vi "Containers by Target.vi"(7 "Target Name":string, 10 "Targets":refnum<vi>[](array[refnum])) -> (1 "Container Names":string[](array[string]), 2 "Container Paths":path[](array[path]), 3 "Target":refnum<vi>)   [LabVIEW 2020, in "Conditum-Tools.lvlib" / "Entity Editor.lvclass"]
uses:
  Entity Editor.lvclass
  Entity Editor.lvclass/Entity Editor.ctl
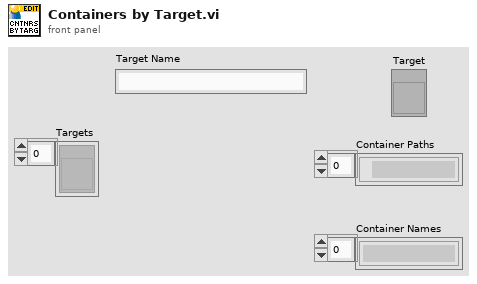
[diagram p1: front panel]
types:
  T1 = enum32{"invalid scope", "public", "private", "protected", "community"}
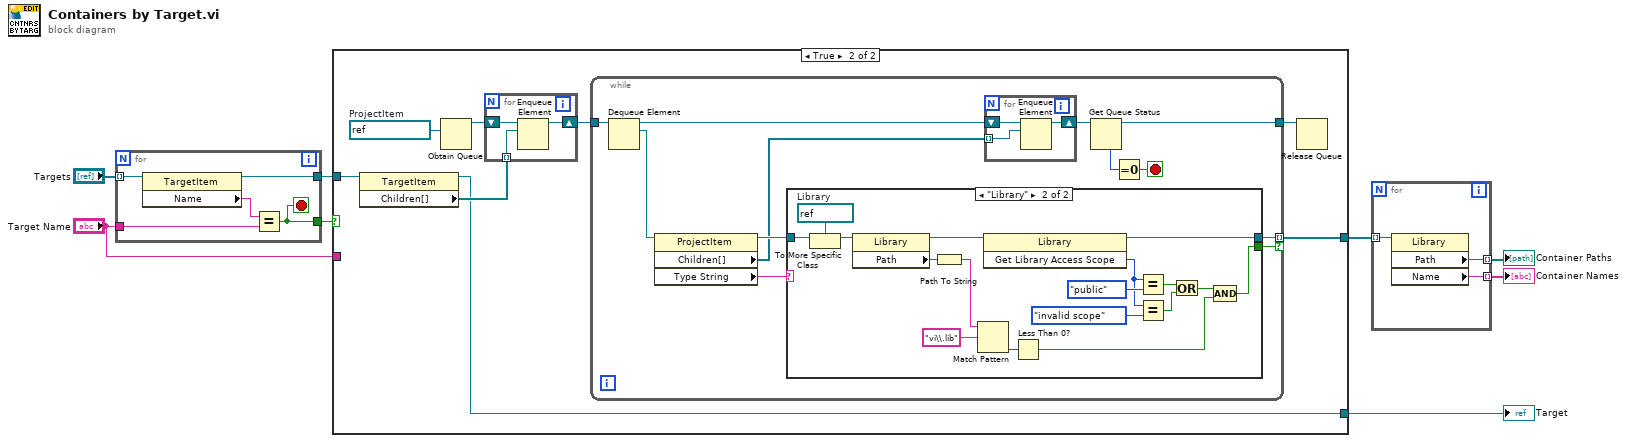
[diagram p0: block diagram]
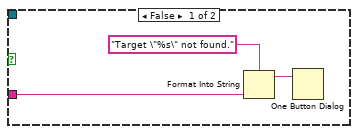
[diagram p2: hidden frame]
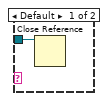
[diagram p3: hidden frame]
diagram:
  n1 = for {
    tunnel: "Targets" -> [w13] mode=indexing
    tunnel: "Target Name" -> [w12]
    tunnel: [w10] -> w6
    tunnel: [w9] -> w7
    stop <- w9 stop-if-true
    n2 = property class="TargetItem"(reference=w13) -> (reference out=w10:refnum<vi>, "Name"=w11:string)  [unwired: 1 in, 1 out]
    n3 = Equal?(x=w11, y=w12) -> (x = y?=w9:bool)
  }
  n4 = case shown="True" w7 {
    tunnel: w6 -> [_ w24]
    tunnel: [_ w18] -> w4
    tunnel: "Target Name" -> [w16 _]
    tunnel: [_ w17] -> w2
    frame False {
      n5 = Format Into String(format string="Target \"%s\" not found.", w16) -> (resulting string=w14:string)  [unwired: 2 in, 1 out]
      n6 = One Button Dialog(message=w14) -> ()  [unwired: 1 in, 1 out]
    }
    frame True {
      w23 = refnum<vi> refnum  # ProjectItem
      n7 = property class="TargetItem"(reference=w24) -> (reference out=w17:refnum<vi>, "Children[]"=w21:refnum<vi>[])  [unwired: 1 in, 1 out]
      n8 = Obtain Queue(element data type=w23) -> (queue out=w22:refnum<queue>)  [unwired: 4 in, 2 out]
      n9 = for {
        shift-right: [w58] -> w20
        shift-left: w22 -> [w60]
        tunnel: w21 -> [w59] mode=indexing
        n10 = Enqueue Element(queue=w60, element=w59) -> (queue out=w58:refnum<queue>)  [unwired: 2 in, 2 out]
      }
      n11 = while {
        tunnel: w20 -> [w36]
        tunnel: [w35] -> w19
        tunnel: [w27] -> w18 mode=indexing if=w26
        stop <- w33 stop-if-true
        n12 = Dequeue Element(queue=w36) -> (queue out=w32:refnum<queue>, element=w30:refnum<vi>)  [unwired: 2 in, 2 out]
        n13 = property class="ProjectItem"(reference=w30) -> (reference out=w28:refnum<vi>, "Children[]"=w25:refnum<vi>[], "Type String"=w29:string)  [unwired: 1 in, 1 out]
        n14 = case shown="\"Library\"" w29 {
          tunnel: w28 -> [w37 w54]
          tunnel: [_ w47] -> w27
          tunnel: [_ w40] -> w26
          frame Default {
            n15 = Close Reference(reference=w37) -> ()  [unwired: 1 in, 1 out]
          }
          frame "Library" {
            w53 = refnum<vi> refnum  # Library
            n16 = To More Specific Class(target class=w53, reference=w54) -> (specific class reference=w46:refnum<vi>)  [unwired: 1 in, 1 out]
            n17 = property class="Library"(reference=w46) -> (reference out=w44:refnum<vi>, "Path"=w43:path)  [unwired: 1 in, 1 out]
            n18 = Path To String(path=w43) -> (string=w42:string)
            n19 = Match Pattern(string=w42, regular expression="vi\\.lib") -> (offset past match=w39:i32)  [unwired: 1 in, 3 out]
            n20 = invoke class="Library" method="Get Library Access Scope"(reference=w44) -> (reference out=w47:refnum<vi>, "Get Library Access Scope"=w50:T1)  [unwired: 2 in, 1 out]
            n21 = Less Than 0?(x=w39) -> (x < 0?=w38:bool)
            n22 = Equal?(x=w50, y=T1."public") -> (x = y?=w49:bool)
            n23 = Equal?(x=w50, y=T1."invalid scope") -> (x = y?=w48:bool)
            n24 = Or(x=w49, y=w48) -> (x .or. y?=w45:bool)
            n25 = Compound Arithmetic op=AND(w45, w38) -> (w40:bool)
          }
        }
        n26 = for {
          shift-right: [w56] -> w31
          shift-left: w32 -> [w57]
          tunnel: w25 -> [w55] mode=indexing
          n27 = Enqueue Element(queue=w57, element=w55) -> (queue out=w56:refnum<queue>)  [unwired: 2 in, 2 out]
        }
        n28 = Get Queue Status(queue=w31) -> (queue out=w35:refnum<queue>, # elements in queue=w34:i32)  [unwired: 2 in, 6 out]
        n29 = Equal To 0?(x=w34) -> (x = 0?=w33:bool)
      }
      n30 = Release Queue(queue=w19) -> ()  [unwired: 2 in, 3 out]
    }
  }
  "Target" <- w2
  n31 = for {
    tunnel: w4 -> [w63] mode=indexing
    tunnel: [w62] -> w3 mode=indexing
    tunnel: [w61] -> w1 mode=indexing
    n32 = property class="Library"(reference=w63) -> ("Path"=w61:path, "Name"=w62:string)  [unwired: 1 in, 2 out]
  }
  "Container Names" <- w3
  "Container Paths" <- w1
